vi "PMOD Example(RT).vi"() -> ()   [LabVIEW 2014]
doc: "The continuous acquisition mode tells the FPGA to acquire points indefinitely until a stop command is issued or until an error is encountered (FIFO overflow, module underflow, and so on). \n\nIn this acquisition mode, explicitly call the appropriate rwfm_ConfigTiming VI and set the host application's data buffer to be many times larger than the read size. The examples use a 10X size by default. If the host application's data buffer fills, then the FPGA experiences a FIFO overflow causing the acquisition to stop."
uses:
  <vilib>/FPGAPlugInAG/sbRIO-9651/niLvFpga_Open_sbRIO-9651.vi
  <vilib>/rvi/interface/common/dynamic/niFpgaDynamicAddResources.vi
  <vilib>/FPGAPlugInAG/Dynamic/niLvFpga_Reset_Dynamic.vi
  <vilib>/FPGAPlugInAG/Dynamic/niLvFpga_Run_Dynamic.vi
  <vilib>/Utility/error.llb/Error Cluster From Error Code.vi
  <vilib>/rvi/errors/niLvFpgaAdjustHostInterfaceError.vi
  <vilib>/FPGAPlugInAG/Dynamic/niLvFpga_Close_Dynamic.vi
  <vilib>/rvi/interface/nirviOpenFPGA/nirviOpenFPGA.xnode
  FPGA Bitfiles/SPIEngineExample_FPGATarget_PMODExample(FPGA_ExF6tyyldTo.lvbitx
  <vilib>/rvi/interface/nirviMethod/nirviMethod.xnode
  <vilib>/rvi/interface/nirviReadWriteControl/nirviReadWriteControl.xnode
  <vilib>/rvi/interface/nirviCloseFPGA/nirviCloseFPGA.xnode
  <vilib>/rvi/interface/Simulation/niFpgaSimulationCallBeginRW.vi
  NiFpgaLv.dll
panel:
  in  "data rate (S/s)":u32
  in  "Voltage Output":u64=3 format="%f"
  in  "SPI PHY Settings":T1={"Divide Value"=20, "Transfer Length (bits)"=32, "CS Asserted Polarity"=FALSE, "Clock Polarity (CPOL)"=FALSE, "Clock Phase (CPHA)"=FALSE, "Lengthen MISO Setup"=FALSE, "Direction Change Bit"=0, "MOSI Starts as Output"=FALSE, "Tristatable MOSI"=FALSE}
  in  "stop":bool
  # "SPI Settings"
  # "Sampling Info"
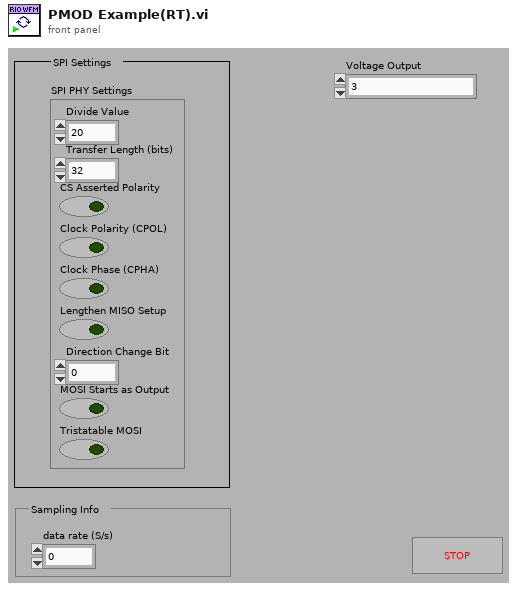
[diagram p1: front panel]
types:
  T1 = cluster{"Divide Value":u8, "Transfer Length (bits)":u8, "CS Asserted Polarity":bool, "Clock Polarity (CPOL)":bool, "Clock Phase (CPHA)":bool, "Lengthen MISO Setup":bool, "Direction Change Bit":u8, "MOSI Starts as Output":bool, "Tristatable MOSI":bool}
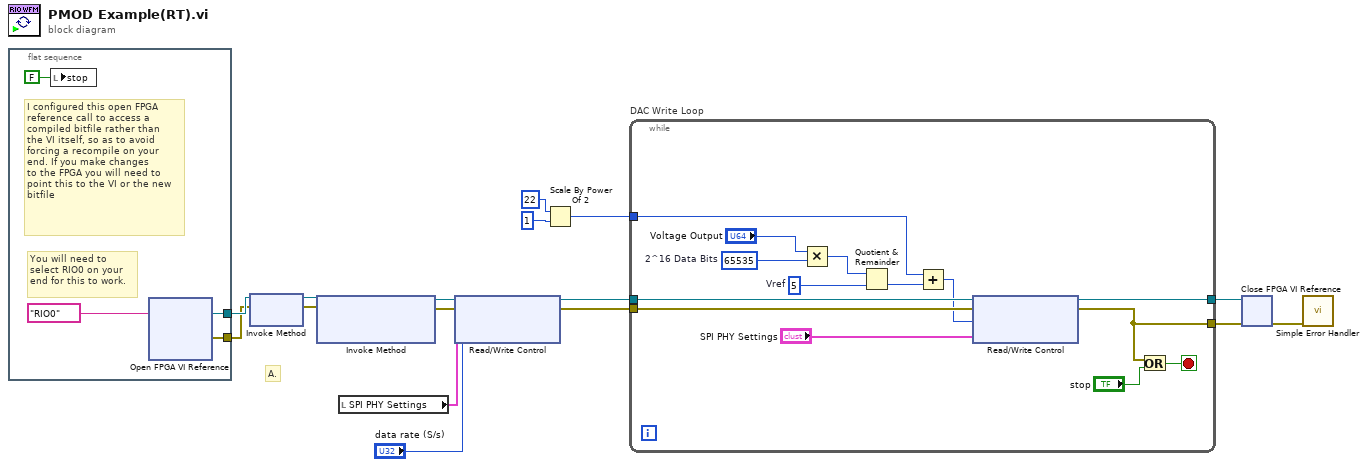
[diagram p0: block diagram]
diagram:
  # "A."
  n1 = flat-sequence {
    tunnel: [w19] -> w16
    tunnel: [w18] -> w15
    frame #0 {
      # "You will need to\nselect RIO0 on your\nend for this to work."
      # "I configured this open FPGA\nreference call to access a\ncompiled bitfile rather than \nthe VI itself, so as to avoid\nforcing a recompile on your\nend. If you make changes\nto the FPGA you will need to\npoint this to the VI or the new\nbitfile"
      n2 = local write "stop"(FALSE ("stop")) -> ()
      n3 = xnode "Open FPGA VI Reference"("resource name"=tag "RIO0") -> ("FPGA VI Reference Out"=w19:refnum<k20>, "error out"=w18:errorcluster)  [unwired: 1 in]
    }
  }
  n4 = xnode "Invoke Method"("FPGA VI Reference In"=w16, "error in"=w15) -> ("FPGA VI Reference Out"=w10:refnum<k20>, "error out"=w9:errorcluster)
  n5 = xnode "Invoke Method"("FPGA VI Reference In"=w10, "error in"=w9) -> ("FPGA VI Reference Out"=w11:refnum<k20>, "error out"=w13:errorcluster)  [unwired: 1 in]
  n6 = local read "SPI PHY Settings"() -> (w3:T1)
  n7 = xnode "Read/Write Control"("FPGA VI Reference In"=w11, "error in"=w13, "SPI PHY Settings"=w3, "data rate (S/s)"="data rate (S/s)") -> ("FPGA VI Reference Out"=w7:refnum<k20>, "error out"=w12:errorcluster)
  n8 = Scale By Power Of 2(n=i16 22, x=u64 1) -> (x*2^n=w4:u64)
  n9 = while "DAC Write Loop" {
    tunnel: w7 -> [w32]
    tunnel: w12 -> [w31]
    tunnel: w4 -> [w28]
    tunnel: [w22] -> w2
    tunnel: [w21] -> w1
    stop <- w34 stop-if-true
    w24 = u64 5  # Vref
    w29 = u64 65535  # 2^16 Data Bits
    n10 = Multiply(x="Voltage Output", y=w29) -> (x*y=w25:u64)
    n11 = Quotient & Remainder(x=w25, y=w24) -> (floor(x/y)=w23:u64)  [unwired: 1 out]
    n12 = Add(x=w28, y=w23) -> (x+y=w26:u64)
    n13 = xnode "Read/Write Control"("FPGA VI Reference In"=w32, "error in"=w31, "Data To ADC"=w26, "SPI PHY Settings"="SPI PHY Settings") -> ("FPGA VI Reference Out"=w22:refnum<k20>, "error out"=w21:errorcluster)
    n14 = Or(x=w21, y="stop") -> (x .or. y?=w34:bool)
  }
  n15 = xnode "Close FPGA VI Reference"("FPGA VI Reference In"=w2, "error in"=w1) -> ("error out"=w14:errorcluster)
  n16 = call <vilib>:"Simple Error Handler.vi"("error in (no error)"=w14) -> ()  [unwired: 1 in, 8 out]
